vi "APPA207.vi"(4 "error in":T13, 7 "Command":T14) -> (0 "error out":T13, 3 "Response":T11)   [LabVIEW 2018]
uses:
  MOKO_LabViewLibrary/MokoLowLevel/MokoLowLovelControl/MLLC_Command.ctl
  MOKO_LabViewLibrary/MokoLowLevel/MokoLowLovelControl/MLLC_Error.ctl
  MOKO_LabViewLibrary/MokoLowLevel/MokoLowLovelControl/MLLC_Mode.ctl
  MOKO_LabViewLibrary/MokoLowLevel/MokoLowLovelControl/MLLC_Response.ctl
  MOKO_LabViewLibrary/MokoLowLevel/MokoLowLovelControl/MLLC_DriverName.ctl
  MOKO_LabViewLibrary/MokoLowLevel/MokoLowLovelControl/MLLC_Request.ctl
  MOKO_LabViewLibrary/MokoLowLevel/MokoLowLovelControl/MLLC_ErrorCode.ctl
  MOKO_LabViewLibrary/MokoLowLevel/MokoLowLovelControl/MLLC_ConnectCluster.ctl
  MOKO_LabViewLibrary/MokoLowLevel/MokoLowLovelControl/MLLC_InterfaceType.ctl
  MOKO_LabViewLibrary/MokoLowLevel/MokoLowLovelControl/MLLC_OpenedSession.ctl
  MOKO_LabViewLibrary/MokoLowLevel/MokoLowLovelControl/MLLC_InterfaceSettings.ctl
  MOKO_LabViewLibrary/MokoLowLevel/MokoLowLovelControl/MLLC_InterfaceKind.ctl
  MOKO_LabViewLibrary/MokoLowLevel/MokoLowLovelControl/MLLC_ResponseInit.ctl
  MOKO_LabViewLibrary/MokoLowLevel/MokoLowLovelControl/MLLC_Rs232Settings.ctl
panel:
  in  "ResponseInit":T1="OK"
  in  "Settings":T7={"Data"={"Connect"={"InterfaceType"=enum."VISA", "OpenedSession"="", "InterfaceSettings"={"Interface"=enum."RS232", "EOS 4 read"=enum."None", "EOS 4 write"=enum."None", "TMO, ms"=1000, "Sett"=variant(cluster{"Baud Rate":u32, "Data Bits":u16, "Parity":u16, "Stop Bits":u16, "Flow Control":u16, "Eho":bool} {"Baud Rate"=75, "Data Bits"=0, "Parity"=0, "Stop Bits"=0, "Flow Control"=0, "Eho"=FALSE})}}}, "Saved Data"=variant}
  in  "Error Code":T8=5475
  in  "Request":T9="UU\u0000\u0000ª"
  in  "Driver Name":T10="APPA207"
  in  "Mode":T12=enum."Check"
  # "APPA207"
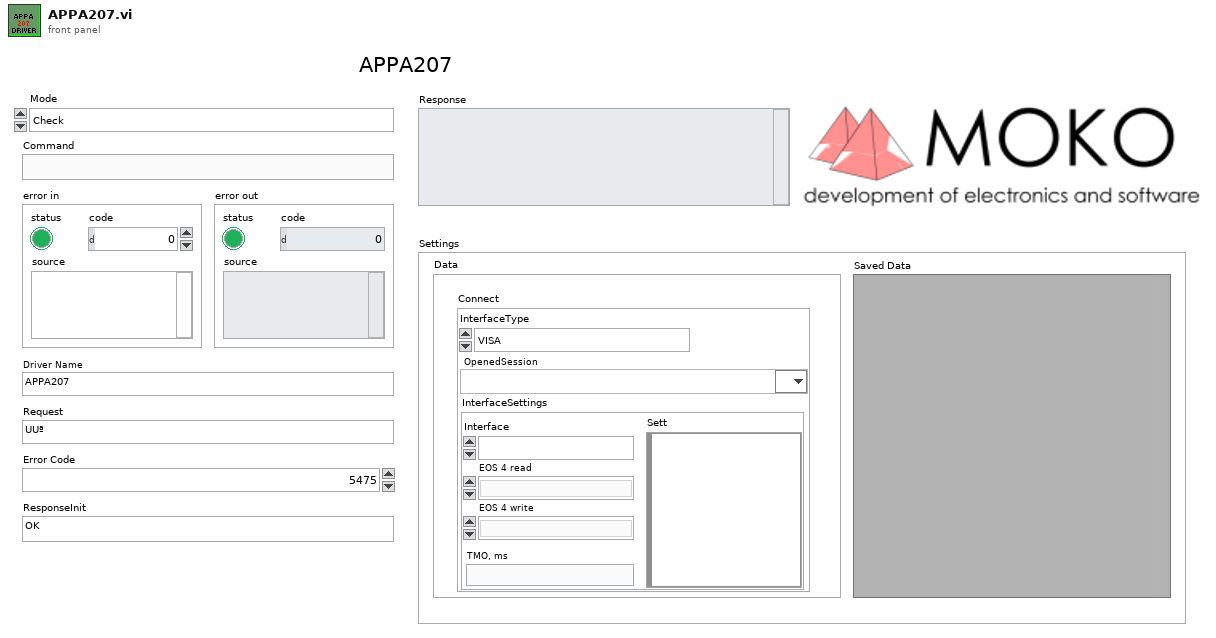
[diagram p1: front panel]
types:
  T1 = typedef "MLLC_ResponseInit.ctl" = string
  T2 = typedef "MLLC_ConnectCluster.ctl" = cluster{"InterfaceType":T3, "OpenedSession":T4, "InterfaceSettings":T5}
  T3 = typedef "MLLC_InterfaceType.ctl" = enum16{"VISA", "Prologix USB-GPIB"}
  T4 = typedef "MLLC_OpenedSession.ctl" = refnum<visa-resource-name>
  T5 = typedef "MLLC_InterfaceSettings.ctl" = cluster{"Interface":T6, "EOS 4 read":enum16{"Default (=EOS 4 write)", "CR (\\r)", "LF (\\n)", "None"}, "EOS 4 write":enum16{"CR+LF (\\r\\n)", "CR (\\r)", "LF (\\n)", "None"}, "TMO, ms":i32, "Sett":variant}
  T6 = typedef "MLLC_InterfaceKind.ctl" = enum16{"RS232", "GPIB", "USB", "Ethernet", "another"}
  T7 = cluster{"Data":cluster{"Connect":T2}, "Saved Data":variant}
  T8 = typedef "MLLC_ErrorCode.ctl" = u32
  T9 = typedef "MLLC_Request.ctl" = string
  T10 = typedef "MLLC_DriverName.ctl" = string
  T11 = typedef "MLLC_Response.ctl" = string
  T12 = typedef "MLLC_Mode.ctl" = enum16{"get", "set", "close", "Init", "Check"}
  T13 = typedef "MLLC_Error.ctl" = errorcluster
  T14 = typedef "MLLC_Command.ctl" = string
  T15 = typedef "MLLC_Rs232Settings.ctl" = cluster{"Baud Rate":u32, "Data Bits":u16, "Parity":u16, "Stop Bits":u16, "Flow Control":u16, "Eho":bool, "Address":dbl}
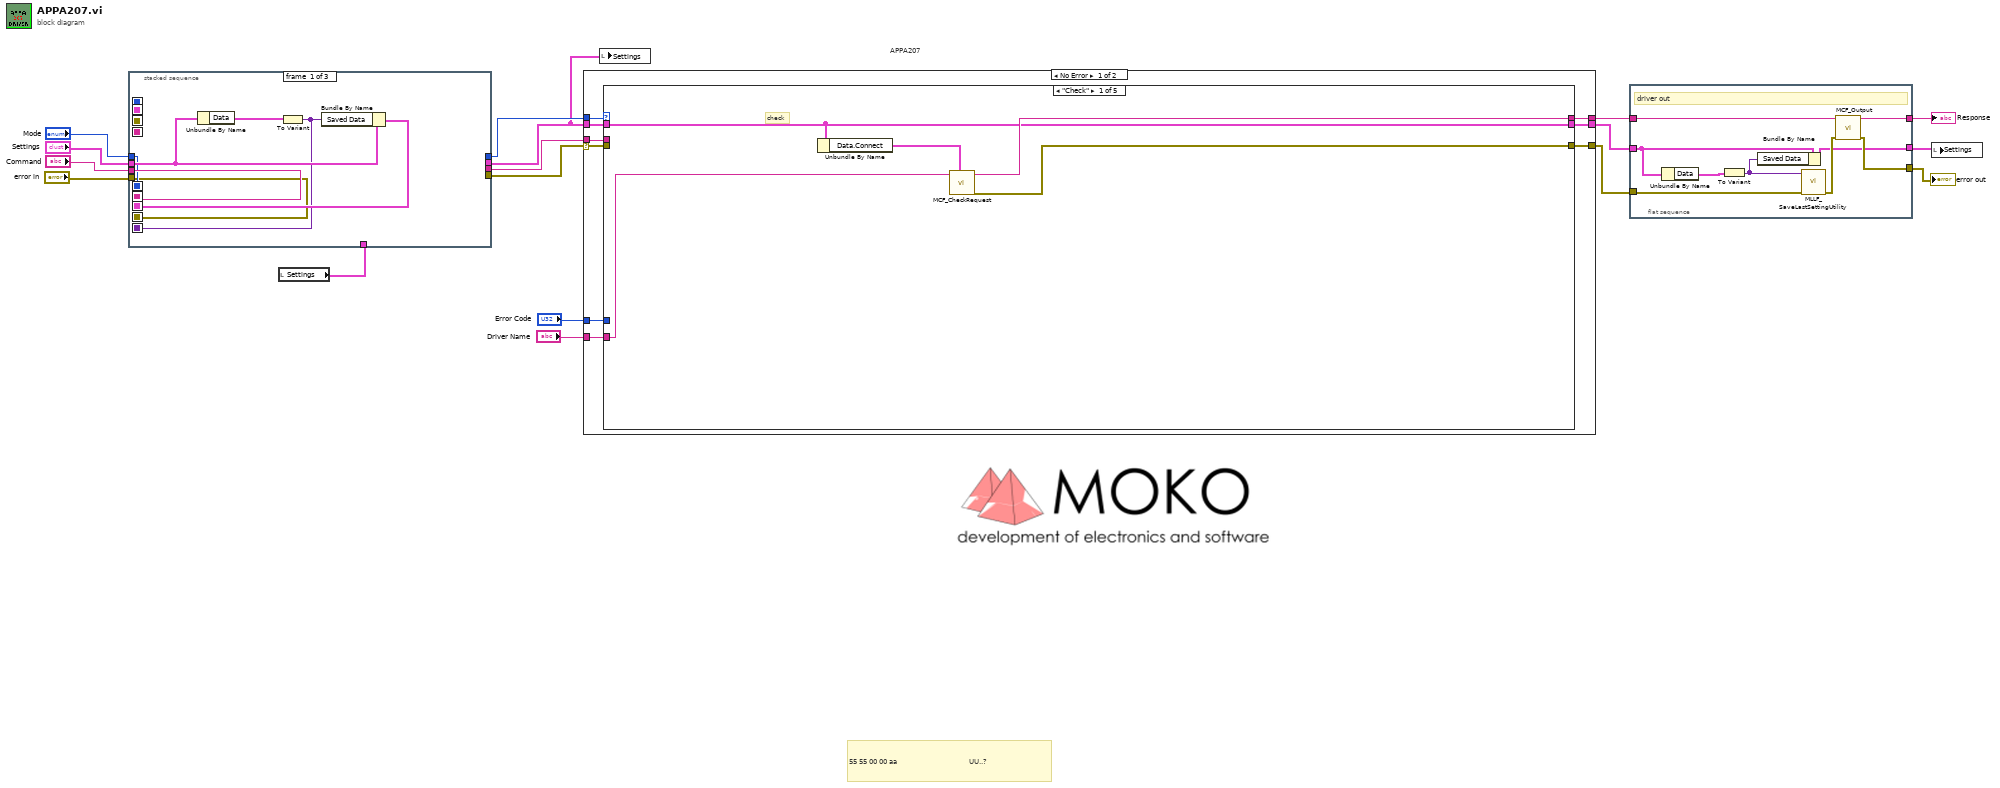
[diagram p0: block diagram]
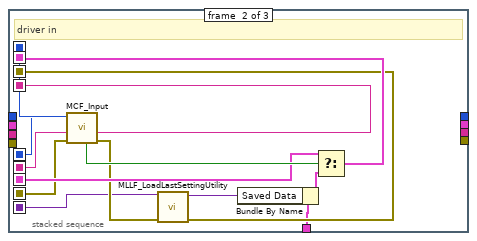
[diagram p2: hidden frame]
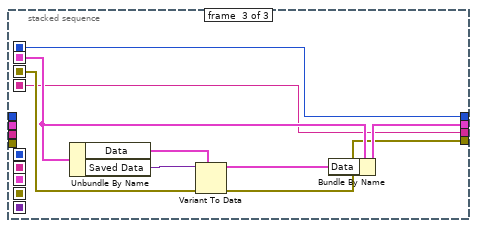
[diagram p3: hidden frame]
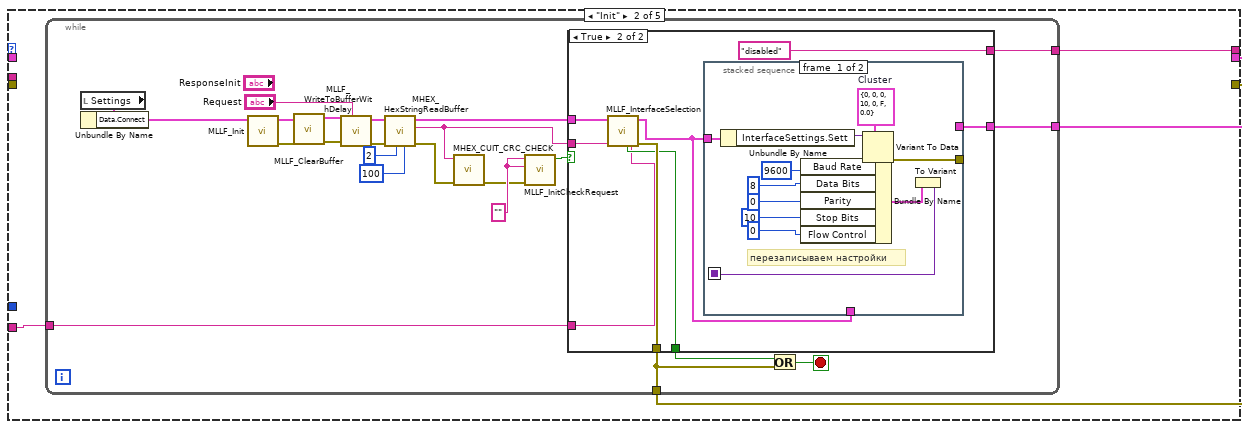
[diagram p4: hidden frame]
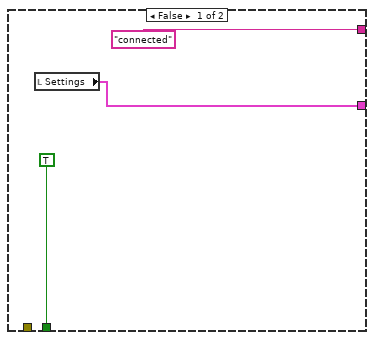
[diagram p5: hidden frame]
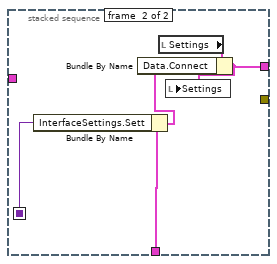
[diagram p6: hidden frame]
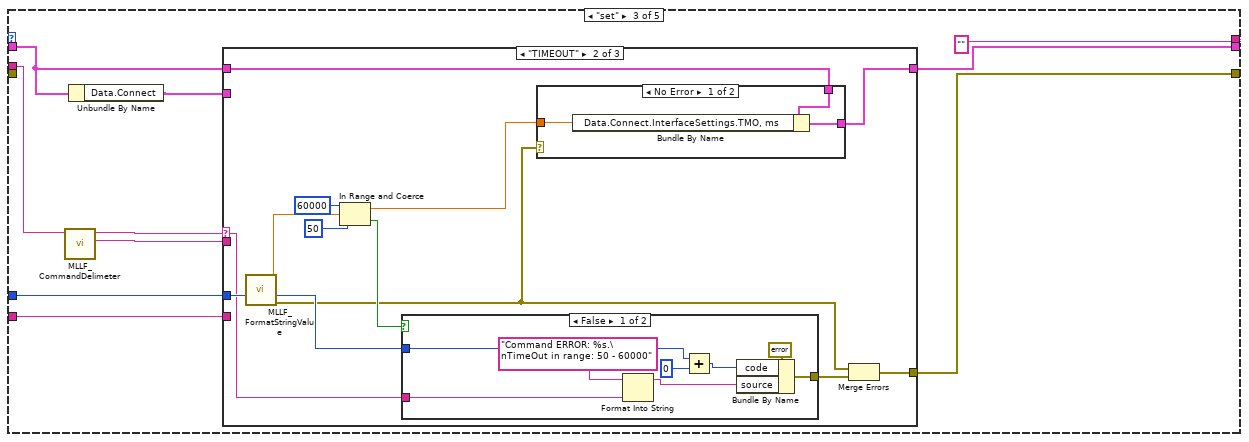
[diagram p7: hidden frame]
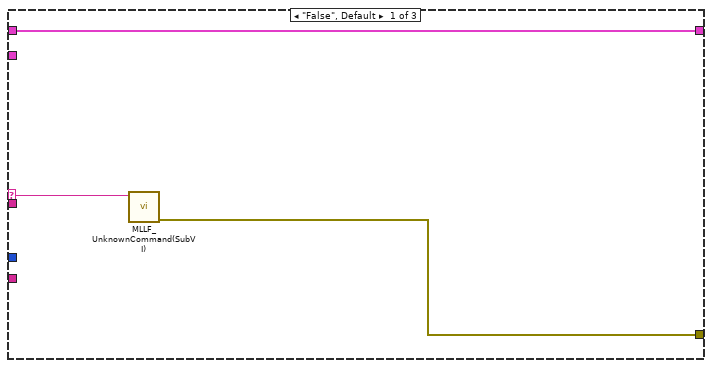
[diagram p8: hidden frame]
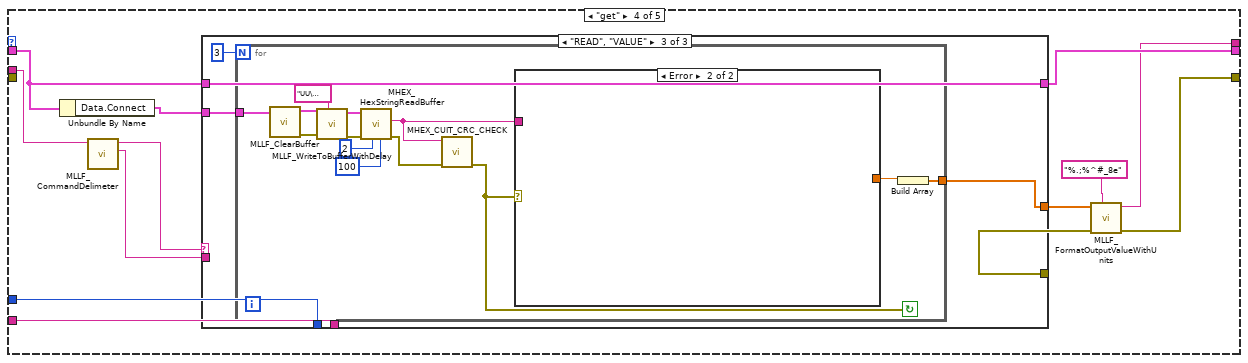
[diagram p12: hidden frame]
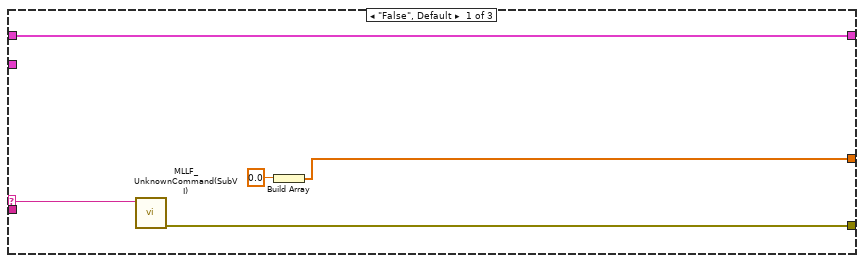
[diagram p13: hidden frame]
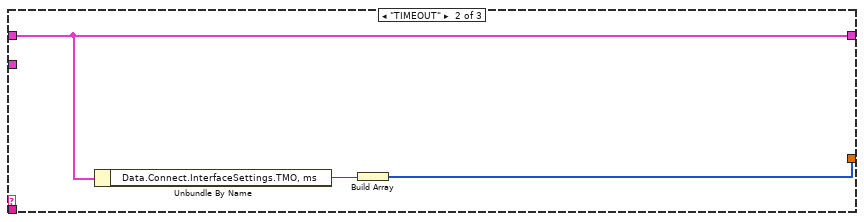
[diagram p14: hidden frame]
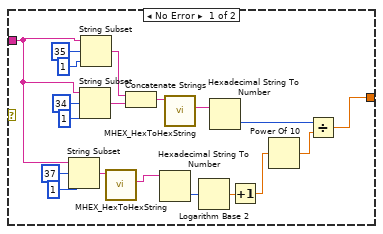
[diagram p15: hidden frame]
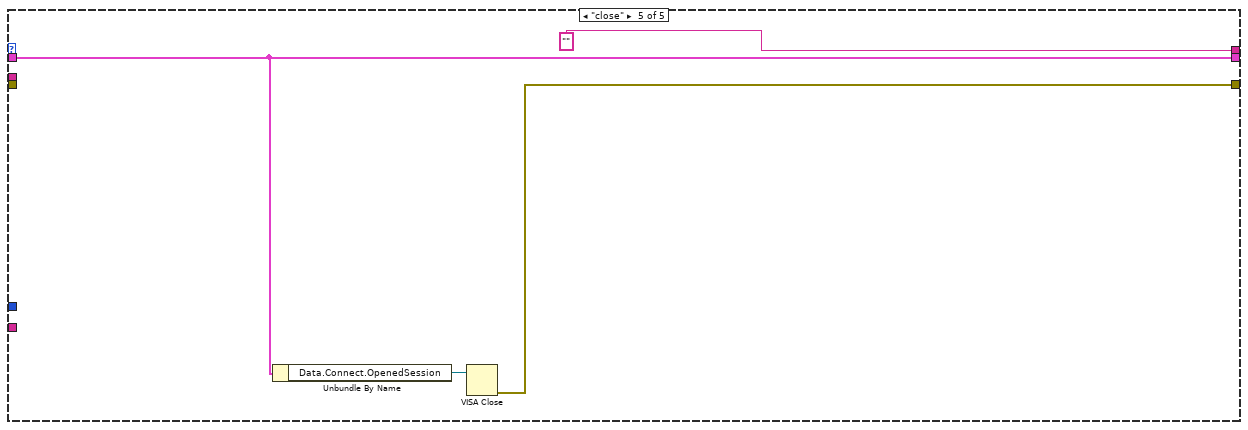
[diagram p16: hidden frame]
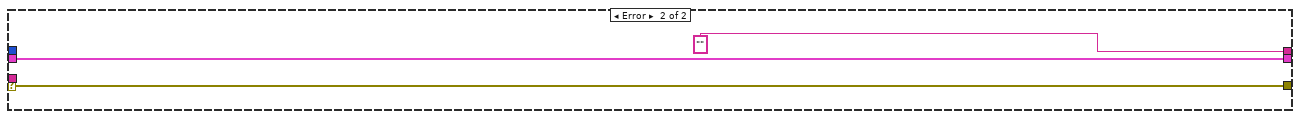
[diagram p17: hidden frame]
diagram:
  # "55 55 00 00 aa                                    UU..?"
  # "APPA207"
  n1 = local read "Settings"() -> (w11:T7)
  n2 = stacked-sequence {
    seq-local: [w20 _ _] -> [_ w36 _]
    seq-local: [w19 _ _] -> [_ w37 _]
    seq-local: [w22 _ _] -> [_ w32 _]
    seq-local: [w18 _ _] -> [_ w31 _]
    seq-local: [w21 _ _] -> [_ w27 _]
    seq-local: [_ w28 _] -> [_ _ w44]
    seq-local: [_ w38 _] -> [_ _ w41]
    seq-local: [_ w35 _] -> [_ _ w40]
    seq-local: [_ w34 _] -> [_ _ w45]
    tunnel: "Command" -> [w20 _ _]
    tunnel: "Mode" -> [w19 _ _]
    tunnel: "error in" -> [w18 _ _]
    tunnel: "Settings" -> [w23 _ _]
    tunnel: w11 -> [_ w26 _]
    tunnel: [_ _ w40] -> w8
    tunnel: [_ _ w43] -> w9
    tunnel: [_ _ w42] -> w7
    tunnel: [_ _ w41] -> w10
    frame #0 {
      n3 = Unbundle By Name(w23) -> ("Data"=w24:cluster{"Connect":T2})
      n4 = To Variant(anything=w24) -> (Variant=w21:variant)
      n5 = Bundle By Name(cluster=w23, "Saved Data"=w21) -> (w22:T7)
    }
    frame #1 {
      # "driver in"
      n6 = call "MCF_Input.vi"("Error In"=w31, "Command in"=w36, "Mode in"=w37) -> ("Error Out"=w30:errorcluster, "Command out"=w35:string, "Mode out"=w38:T12, "Boolean"=w33:bool)  [unwired: 5 in]
      n7 = call "MLLF_LoadLastSettingUtility.vi"("Error In"=w30, "Save data in"=w27) -> ("Error Out"=w28:errorcluster, "Save data out"=w25:variant)  [unwired: 8 in]
      n8 = Bundle By Name(cluster=w26, "Saved Data"=w25) -> (w29:T7)
      n9 = Select(t=w32, s=w33, f=w29) -> (s? t:f=w34:T7)
    }
    frame #2 {
      n10 = Unbundle By Name(w45) -> ("Data"=w46:cluster{"Connect":T2}, "Saved Data"=w39:variant)
      n11 = Variant To Data(error in=w44, type=w46, Variant=w39) -> (data=w47:cluster{"Connect":T2}, error out=w42:errorcluster)
      n12 = Bundle By Name(cluster=w45, "Data"=w47) -> (w43:T7)
    }
  }
  n13 = case shown="No Error" w7 {
    selector: w7 -> [w52 w218]
    tunnel: [w54 w218] -> w4
    tunnel: w10 -> [w56 _]
    tunnel: [w55 "" ("String")] -> w6
    tunnel: w8 -> [w53 _]
    tunnel: w9 -> [w49 w217]
    tunnel: "Error Code" -> [w51 _]
    tunnel: "Driver Name" -> [w50 _]
    tunnel: [w48 w217] -> w5
    frame No Error {
      n14 = case shown="\"Check\"" w56 {
        tunnel: [w60 w65 "" ("String") w160 "" ("String")] -> w55
        tunnel: [w61 w63 w117 w161 w214] -> w54
        tunnel: w53 -> [_ _ w120 w159 _]
        tunnel: w52 -> [_ _ _ _ _]
        tunnel: w51 -> [_ _ w126 w166 _]
        tunnel: w50 -> [w59 w62 w123 w165 _]
        tunnel: w49 -> [w58 _ w125 w156 w213]
        tunnel: [w58 w64 w124 w167 w213] -> w48
        frame "Check" {
          # "check"
          n15 = Unbundle By Name(w58) -> ("Data.Connect"=w57:T2)
          n16 = call "MCF_CheckRequest.vi"("Permanent data.Connect"=w57, "Driver Name"=w59) -> ("Error Out"=w61:errorcluster, "Output String"=w60:string)  [unwired: 8 in]
        }
        frame "Init" {
          n17 = while {
            tunnel: [w84] -> w63
            tunnel: [w82] -> w65
            tunnel: [w81] -> w64
            tunnel: w62 -> [w67]
            stop <- w83 stop-if-true
            w70 = ""
            n18 = local read "Settings"() -> (w88:T7)
            n19 = Unbundle By Name(w88) -> ("Data.Connect"=w86:T2)
            n20 = call "MLLF_Init.vi"("DriverConnect in"=w86) -> ("Error Out"=w75:errorcluster, "DriverConnect out"=w76:T2)  [unwired: 7 in]
            n21 = call "MLLF_ClearBuffer.vi"("Error In"=w75, "DriverConnect in"=w76) -> ("Error Out"=w73:errorcluster, "DriverConnect out"=w74:T2)  [unwired: 6 in, 1 out]
            n22 = call "MLLF_WriteToBufferWithDelay.vi"("Command"="Request", "Error In"=w73, "DriverConnect in"=w74) -> ("Error Out"=w78:errorcluster, "DriverConnect out"=w79:T2)  [unwired: 7 in]
            n23 = call "MHEX_HexStringReadBuffer.vi"("byte count"=u32 100, "length (rest)"=2, "error in"=w78, "DriverConnect in"=w79) -> ("error out"=w68:T13, "String from device out"=w66:string, "DriverConnect out"=w77:T2)  [unwired: 4 in, 1 out]
            n24 = call "MHEX_CUIT_CRC_CHECK.vi"("Error In"=w68, "string in"=w66) -> ("Error Out"=w69:errorcluster)  [unwired: 9 in]
            n25 = call "MLLF_InitCheckRequest.vi"("error in (no error)"=w69, "Answer"=w70, "Response Init"=w70) -> ("Design"=w80:bool)  [unwired: 5 in, 3 out]
            n26 = case shown="True" w80 {
              tunnel: w77 -> [_ w99]
              tunnel: [TRUE w96] -> w85
              tunnel: [_ w98] -> w84
              tunnel: ["connected" "disabled"] -> w82
              tunnel: [w89 w94] -> w81
              tunnel: w67 -> [_ w93]
              tunnel: w66 -> [_ w92]
              frame False {
                n27 = local read "Settings"() -> (w89:T7)
              }
              frame True {
                n28 = call "MLLF_InterfaceSelection.vi"("Driver Name"=w93, "Answer:"=w92, "DriverConnect in"=w99) -> ("error out"=w98:T13, "DriverConnect out"=w95:T2, "stop init?"=w96:bool)  [unwired: 4 in, 2 out]
                n29 = stacked-sequence {
                  seq-local: [w101 _] -> [_ w115]
                  tunnel: w95 -> [w102 _]
                  tunnel: w95 -> [_ w114]
                  tunnel: [_ w112] -> w94
                  tunnel: [w100 _] -> _
                  frame #0 {
                    w105 = T15 {"Baud Rate"=0, "Data Bits"=0, "Parity"=0, "Stop Bits"=10, "Flow Control"=0, "Eho"=FALSE, "Address"=0.0}  # Cluster
                    # "перезаписываем настройки"
                    n30 = Unbundle By Name(w102) -> ("InterfaceSettings.Sett"=w104:variant)
                    n31 = Variant To Data(type=w105, Variant=w104) -> (data=w106:T15, error out=w100:errorcluster)  [unwired: 1 in]
                    n32 = Bundle By Name(cluster=w106, "Baud Rate"=u32 9600, "Data Bits"=u16 8 ("Serial Settings:Data Bits"), "Parity"=u16 0 ("Serial Settings:Parity"), "Stop Bits"=u16 10 ("Serial Settings:Stop Bits"), "Flow Control"=u16 0 ("Serial Settings:Flow Control")) -> (w111:T15)
                    n33 = To Variant(anything=w111) -> (Variant=w101:variant)
                  }
                  frame #1 {
                    n34 = Bundle By Name(cluster=w114, "InterfaceSettings.Sett"=w115) -> (w113:T2)
                    n35 = local read "Settings"() -> (w116:T7)
                    n36 = Bundle By Name(cluster=w116, "Data.Connect"=w113) -> (w112:T7)
                    n37 = local write "Settings"(w112) -> ()
                  }
                }
              }
            }
            n38 = Or(x=w85, y=w84) -> (x .or. y?=w83:bool)
          }
        }
        frame "set" {
          n39 = call "MLLF_CommandDelimeter.vi"("command with param"=w120) -> ("param 1"=w118:string, "command"=w119:string)  [unwired: 6 in, 3 out]
          n40 = Unbundle By Name(w125) -> ("Data.Connect"=w121:T2)
          n41 = case shown="\"TIMEOUT\"" w119 {
            selector: w119 -> [w128 w130 _]
            tunnel: w118 -> [_ _ _]
            tunnel: [w127 w135 _] -> w117
            tunnel: w126 -> [_ w136 _]
            tunnel: w125 -> [w129 w140 w154]
            tunnel: [w129 w141 w154] -> w124
            tunnel: w121 -> [_ _ _]
            tunnel: w123 -> [_ _ _]
            frame "False", Default {
              n42 = call "MLLF_UnknownCommand(SubVI).vi"("Unknown command"=w128) -> ("error out"=w127:errorcluster)  [unwired: 10 in]
            }
            frame "TIMEOUT" {
              n43 = call "MLLF_FormatStringValue.vi"() -> ("error out"=w131:T13, "number"=w132:dbl)  [unwired: 9 in, 1 out]
              n44 = In Range and Coerce(upper limit=60000, x=w132, lower limit=50) -> (coerced(x)=w137:dbl, In Range?=w133:bool)
              n45 = case shown="False" w133 {
                tunnel: [w148 _] -> w134
                tunnel: w136 -> [w147 _]
                tunnel: w130 -> [w146 _]
                frame False {
                  n46 = Format Into String(format string="Command ERROR: %s.\nTimeOut in range: 50 - 60000", w146) -> (resulting string=w150:string)  [unwired: 2 in, 1 out]
                  n47 = Add(x=w147, y=0) -> (x+y=w151:T8)
                  n48 = Bundle By Name(cluster=errorcluster {"status"=TRUE, "code"=0, "source"=""} ("error out"), "code"=w151, "source"=w150) -> (w148:errorcluster)
                }
                frame True {
                }
              }
              n49 = case shown="No Error" w131 {
                tunnel: [w144 w145] -> w141
                tunnel: w140 -> [w143 w145]
                tunnel: w137 -> [w142 _]
                frame No Error {
                  n50 = Bundle By Name(cluster=w143, "Data.Connect.InterfaceSettings.TMO, ms"=w142) -> (w144:T7)
                }
                frame Error {
                }
              }
              n51 = Merge Errors(w131, w134) -> (w135:errorcluster)
            }
            frame "<----MAIN FUNCTIONS---->" {
            }
          }
        }
        frame "get" {
          n52 = Unbundle By Name(w156) -> ("Data.Connect"=w155:T2)
          n53 = call "MLLF_CommandDelimeter.vi"("command with param"=w159) -> ("param 1"=w157:string, "command"=w158:string)  [unwired: 6 in, 3 out]
          n54 = case shown="\"READ\", \"VALUE\"" w158 {
            selector: w158 -> [w169 _ _]
            tunnel: [w168 _ _] -> w164
            tunnel: w166 -> [_ _ _]
            tunnel: [w172 w175 w178] -> w167
            tunnel: w156 -> [w172 w175 w178]
            tunnel: [w170 w173 w176] -> w163
            tunnel: w165 -> [_ _ _]
            tunnel: w157 -> [_ _ _]
            tunnel: w155 -> [_ _ w179]
            frame "False", Default {
              n55 = call "MLLF_UnknownCommand(SubVI).vi"("Unknown command"=w169) -> ("error out"=w168:errorcluster)  [unwired: 10 in]
              n56 = Build Array(0.0 ("TimeOut")) -> (w170:dbl[])
            }
            frame "TIMEOUT" {
              n57 = Unbundle By Name(w175) -> ("Data.Connect.InterfaceSettings.TMO, ms"=w174:i32)
              n58 = Build Array(w174) -> (w173:i32[])
            }
            frame "READ", "VALUE" {
              n59 = for {
                N: 3 -> [_]
                tunnel: w179 -> [w185]
                tunnel: [w180] -> w176
                stop <- w182 continue-if-true
                n60 = call "MLLF_ClearBuffer.vi"("DriverConnect in"=w185) -> ("Error Out"=w188:errorcluster, "DriverConnect out"=w189:T2)  [unwired: 7 in, 1 out]
                n61 = call "MLLF_WriteToBufferWithDelay.vi"("Command"=T9 "UU\u0000\u0000ª" ("Request 2"), "Error In"=w188, "DriverConnect in"=w189) -> ("Error Out"=w190:errorcluster, "DriverConnect out"=w191:T2)  [unwired: 7 in]
                n62 = call "MHEX_HexStringReadBuffer.vi"("byte count"=u32 100, "length (rest)"=2, "error in"=w190, "DriverConnect in"=w191) -> ("error out"=w183:T13, "String from device out"=w184:string)  [unwired: 4 in, 2 out]
                n63 = call "MHEX_CUIT_CRC_CHECK.vi"("Error In"=w183, "string in"=w184) -> ("Error Out"=w182:errorcluster)  [unwired: 9 in]
                n64 = case shown="Error" w182 {
                  tunnel: w184 -> [w205 _]
                  tunnel: [w193 _] -> w181
                  frame No Error {
                    n65 = String Subset(string=w205, offset (0)=37, length (rest)=1 ("length (rest)")) -> (substring=w200:string)
                    n66 = String Subset(string=w205, offset (0)=34, length (rest)=1 ("length (rest)")) -> (substring=w203:string)
                    n67 = String Subset(string=w205, offset (0)=35, length (rest)=1 ("length (rest)")) -> (substring=w204:string)
                    n68 = call "MHEX_HexToHexString.vi"("STRING HEX"=w200) -> ("Without space"=w199:string)  [unwired: 8 in, 2 out]
                    n69 = Concatenate Strings(w204, w203) -> (w202:string)
                    n70 = Hexadecimal String To Number(string=w199) -> (number=w198:u32)  [unwired: 2 in, 1 out]
                    n71 = call "MHEX_HexToHexString.vi"("STRING HEX"=w202) -> ("Without space"=w201:string)  [unwired: 8 in, 2 out]
                    n72 = Logarithm Base 2(1:w198) -> (0:w197:dbl)
                    n73 = Hexadecimal String To Number(string=w201) -> (number=w195:u32)  [unwired: 2 in, 1 out]
                    n74 = Increment(x=w197) -> (x+1=w196:dbl)
                    n75 = Power Of 10(x=w196) -> (10^x=w194:dbl)
                    n76 = Divide(x=w195, y=w194) -> (x/y=w193:dbl)
                  }
                  frame Error {
                  }
                }
                n77 = Build Array(w181) -> (w180:dbl[])
              }
            }
          }
          n78 = call "MLLF_FormatOutputValueWithUnits.vi"("Format"="%.;%^#_8e" ("format string"), "error in"=w164, "ValuesIn"=w163) -> ("error out"=w161:T13, "Result string"=w160:T14)  [unwired: 7 in]
        }
        frame "close" {
          n79 = Unbundle By Name(w213) -> ("Data.Connect.OpenedSession"=w215:T4)
          n80 = VISA Close(VISA resource name=w215) -> (error out=w214:errorcluster)  [unwired: 1 in]
        }
      }
    }
    frame Error {
    }
  }
  n81 = local write "Settings"(w9) -> ()
  n82 = flat-sequence {
    tunnel: [w227] -> w1
    tunnel: [w226] -> w3
    tunnel: w6 -> [w225]
    tunnel: w4 -> [w224]
    tunnel: w5 -> [w220]
    tunnel: [w222] -> w2
    frame #0 {
      # "driver out"
      n83 = Unbundle By Name(w220) -> ("Data"=w219:cluster{"Connect":T2})
      n84 = To Variant(anything=w219) -> (Variant=w221:variant)
      n85 = Bundle By Name(cluster=w220, "Saved Data"=w221) -> (w222:T7)
      n86 = call "MLLF_SaveLastSettingUtility.vi"("error in"=w224, "Saved Data"=w221) -> ("error out"=w223:T13)  [unwired: 8 in, 1 out]
      n87 = call "MCF_Output.vi"("Error In"=w223, "Input"=w225) -> ("Error Out"=w226:errorcluster, "Output"=w227:string)  [unwired: 8 in]
    }
  }
  n88 = local write "Settings"(w2) -> ()
  "error out" <- w3
  "Response" <- w1
